vi "TimeInterpPose2d_Clear.vi"(11 "in TimeInterpPose":T1 {"Pose"."ROTATION"."SIN" format="%13.4f"; "Pose"."ROTATION"."COS" format="%13.4f"; "Pose"."ROTATION"."VALUE" format="%13.4f"; "Pose"."TRANSLATION"."Y" format="%14.3f"; "Pose"."TRANSLATION"."X" format="%14.3f"}) -> (3 "out TimeInterpPose":T1 {"Pose"."ROTATION"."SIN" format="%13.4f"; "Pose"."ROTATION"."COS" format="%13.4f"; "Pose"."ROTATION"."VALUE" format="%13.4f"; "Pose"."TRANSLATION"."Y" format="%14.3f"; "Pose"."TRANSLATION"."X" format="%14.3f"})   [LabVIEW 2019, in "Trajectory_Library.lvlib"]
doc: "Removes all samples from the history buffer.\n\nInputs:\n - In TimeInterpPose2d -- Input data cluster.\n\nOutputs:\n - Out TimeInterpPose2d -- Updated data cluster."
uses:
  Trajectory_Library.lvlib
  TypeDef/TIME_INTERPOLATABLE_POSE2D.ctl
  POSE2D.ctl
  TRANSLATION2D.ctl
  ROTATION2D.ctl
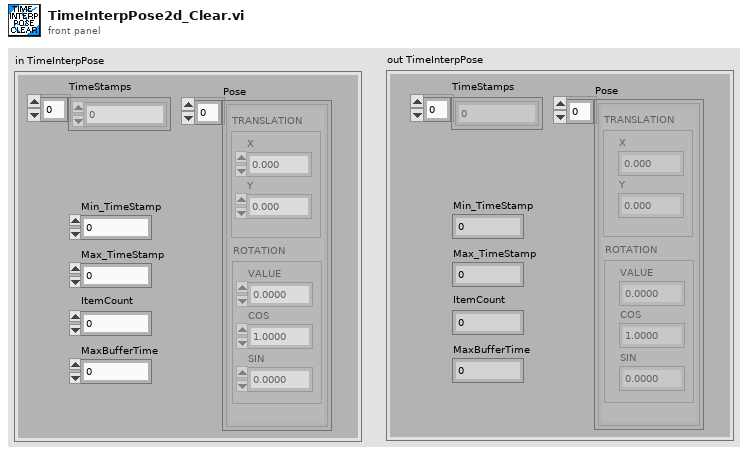
[diagram p1: front panel]
types:
  T1 = typedef "Trajectory_Library.lvlib/TIME_INTERPOLATABLE_POSE2D.ctl" = cluster{"TimeStamps":dbl[], "Pose":T2[], "Min_TimeStamp":dbl, "Max_TimeStamp":dbl, "ItemCount":i32, "MaxBufferTime":dbl}
  T2 = typedef "Trajectory_Library.lvlib/POSE2D.ctl" = cluster{"TRANSLATION":T3, "ROTATION":T4}
  T3 = typedef "Trajectory_Library.lvlib/TRANSLATION2D.ctl" = cluster{"X":dbl, "Y":dbl}
  T4 = typedef "Trajectory_Library.lvlib/ROTATION2D.ctl" = cluster{"VALUE":dbl, "COS":dbl, "SIN":dbl}
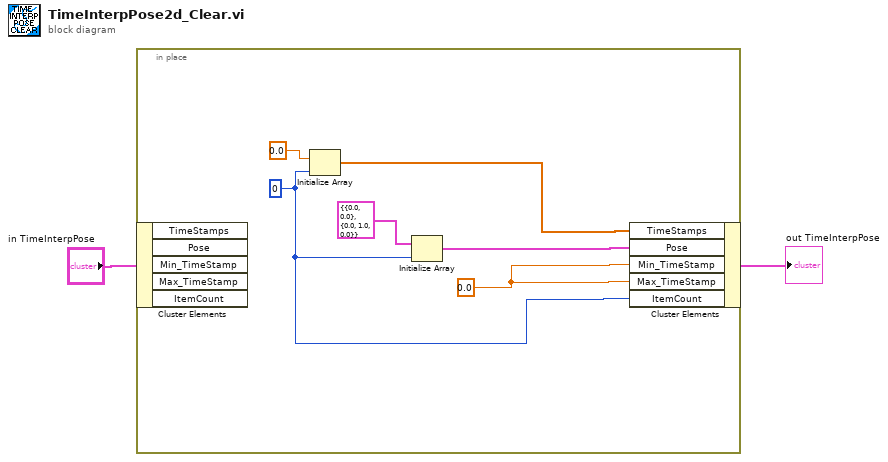
[diagram p0: block diagram]
diagram:
  n1 = in-place {
    w4 = 0.0 ("X")
    w3 = 0 ("dimension size")
    n2 = in-place-cluster #1("in TimeInterpPose") -> ()  [unwired: 5 out]
    n3 = Initialize Array(0.0 ("element"), w3) -> (w6:dbl[])
    n4 = Initialize Array(T2 {"TRANSLATION"={"X"=0.0, "Y"=0.0}, "ROTATION"={"VALUE"=0.0, "COS"=1.0, "SIN"=0.0}} ("POSE"), w3) -> (w5:T2[])
    n5 = in-place-cluster #1("TimeStamps"=w6, "Pose"=w5, "Min_TimeStamp"=w4, "Max_TimeStamp"=w4, "ItemCount"=w3) -> (→"out TimeInterpPose":T1)
  }
